vi "Get_ADAM_averages_client.vi"(6 "No of averages":i32=1, 7 "All Active Channels":bool, 9 "End time":dbl, 10 "Start time":dbl, 11 "ADAM Ch Names":string[](array[string])) -> (1 "Values":string[][](array[string]), 2 "Comments":string[](array[string]), 3 "Titles":string[](array[string]), 4 "Messages":string, 5 "DBL values":dbl[][](array[numeric]) format="%.2f")   [LabVIEW 2017]
doc: "This is an example of using features of the VI Server as a client. It shows how you might browse from one or more applications that may be exporting data from one or more data stations. \n\nThe example shows how to query a server for its list of exported VIs, how to get references to the VIs, and how call them with the Call By Reference function."
uses:
  Anemometry/Anemometry Sub Vis/Controls/Global_mode.ctl
  Sub VIs/ADAM Controls/Channel_names.ctl
  Anemometry/Anemometry Sub Vis/Globals/Preference_global.vi
panel:
  in  "vi type":refnum<vi>
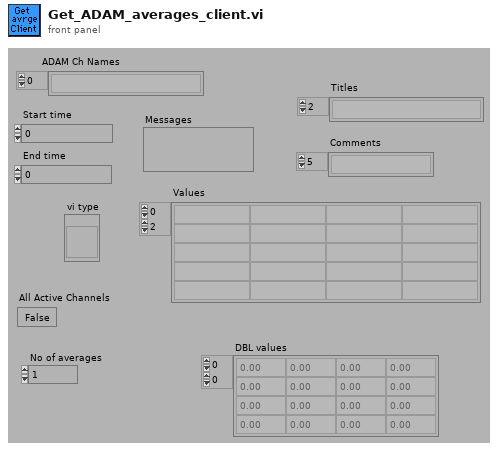
[diagram p1: front panel]
types:
  T1 = typedef "Global_mode.ctl" = enum16{"Read Global", "Load Global From File", "Write Global to File"}
  T2 = typedef "Channel_names.ctl" = enum16{"Active Only", "Active + Off", "All Channels"}
  T3 = typedef "Server_Comms.ctl" = enum16{"Server Link Healthy", "Do Not Link To Server"}
  T4 = typedef "Update_scan_value.ctl" = cluster{"Channel Name":string, "New Value":dbl}
  T5 = typedef "Ch_description_ADAM.ctl" = cluster{"Ch Name":string, "Type":T6, "Function":T7, "Ch State":T8, "Calibration type":T9, "A":dbl, "B":dbl, "C":dbl, "D":dbl, "Comments":string, "Address":T10, "String":string, "Duty":u16}
  T6 = typedef "Module_type_ADAM.ctl" = string
  T7 = typedef "Function_ADAM.ctl" = enum16{"Analogue Input", "Digital Input", "Event counter", "Event rate", "Analogue Output", "Digital Output", "Relay Output"}
  T8 = typedef "Channel_State.ctl" = enum16{"On", "Off", "Always On", "Always Off"}
  T9 = typedef "Calib_type_ADAM.ctl" = string
  T10 = typedef "Address.ctl" = cluster{"Main":i32, "Ch.":i32, "Sub":i32, "Port Name":string}
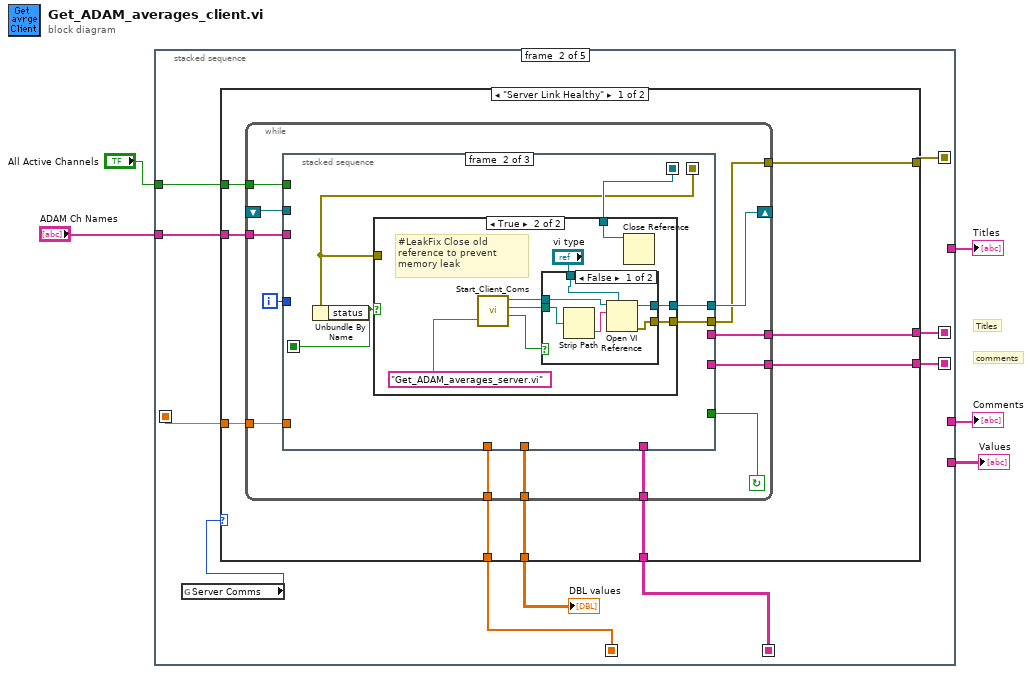
[diagram p0: block diagram]
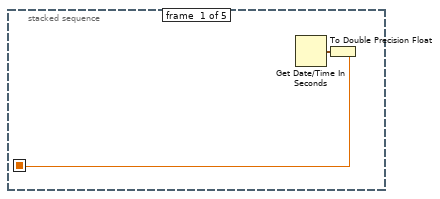
[diagram p2: hidden frame]
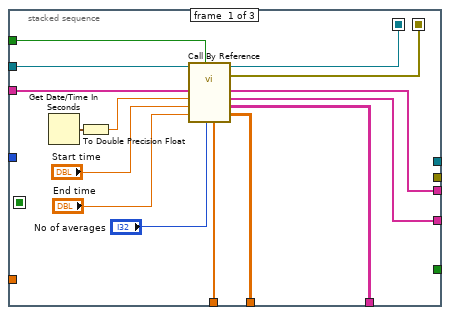
[diagram p3: hidden frame]
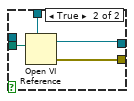
[diagram p5: hidden frame]
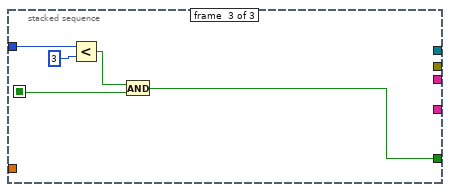
[diagram p6: hidden frame]
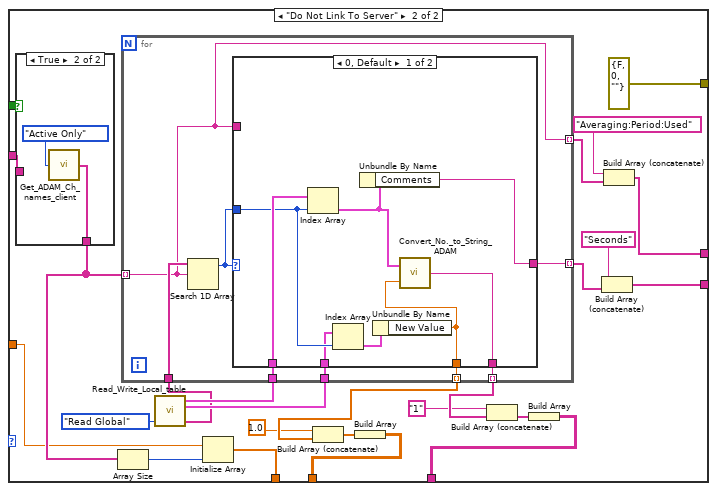
[diagram p7: hidden frame]
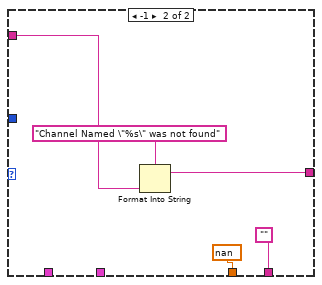
[diagram p9: hidden frame]
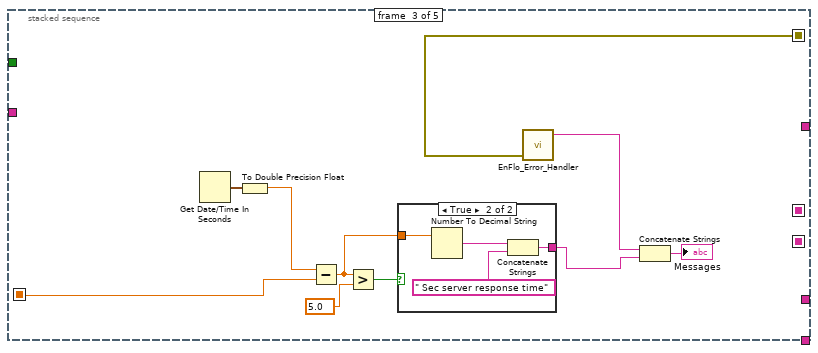
[diagram p10: hidden frame]
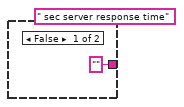
[diagram p11: hidden frame]
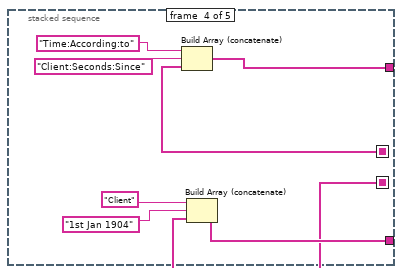
[diagram p12: hidden frame]
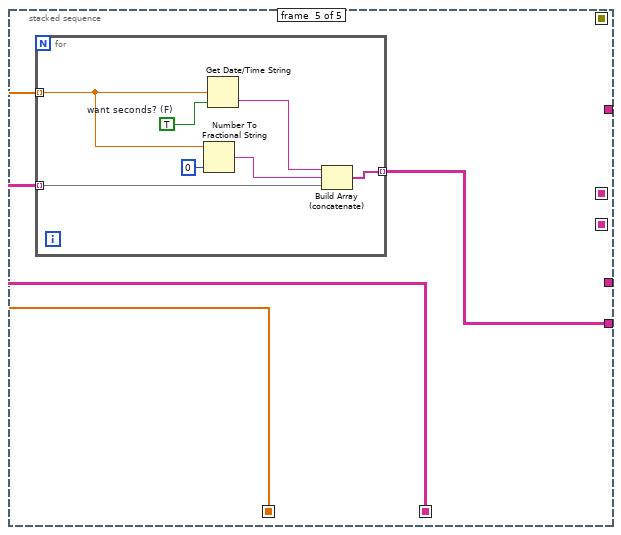
[diagram p13: hidden frame]
diagram:
  # "comments"
  # "Titles"
  n1 = stacked-sequence {
    seq-local: [_ w17 _ _ _] -> [_ _ _ w156 _]
    seq-local: [_ w8 _ _ _] -> [_ _ _ w149 _]
    seq-local: [_ w16 _ _ _] -> [_ _ _ _ w158]
    seq-local: [w7 _ _ _ _] -> [_ w15 w141 _ _]
    seq-local: [_ w14 _ _ _] -> [_ _ _ _ w159]
    seq-local: [_ w13 _ _ _] -> [_ _ w136 _ _]
    tunnel: [_ _ _ w154 _] -> w5
    tunnel: [_ _ _ w155 _] -> w4
    tunnel: [_ _ _ _ w157] -> w3
    tunnel: "ADAM Ch Names" -> [_ w10 _ _ _]
    tunnel: "All Active Channels" -> [_ w9 _ _ _]
    frame #0 {
      n2 = Get Date/Time In Seconds() -> (seconds since 1Jan1904=w6:timestamp)
      n3 = To Double Precision Float(number=w6) -> (double precision float=w7:dbl)
    }
    frame #1 {
      n4 = global read "Preference_global.vi" "Server Comms"() -> (w12:T3)
      n5 = case shown="\"Server Link Healthy\"" w12 {
        tunnel: [w26 w91] -> w17
        tunnel: [w25 w99] -> w16
        tunnel: w15 -> [w24 w89]
        tunnel: [w23 w105] -> w14
        tunnel: [w22 errorcluster {"status"=FALSE, "code"=0, "source"=""}] -> w13
        tunnel: [w21 w85] -> w11
        tunnel: w10 -> [w20 w100]
        tunnel: w9 -> [w19 w103]
        tunnel: [w18 w90] -> w8
        frame "Server Link Healthy" {
          n6 = while {
            tunnel: [w30] -> w22
            shift-left: _ -> [w34]
            shift-right: [w33] -> _
            tunnel: [w35] -> w23
            tunnel: w24 -> [w36]
            tunnel: [w37] -> w25
            tunnel: [w38] -> w18
            tunnel: [w39] -> w26
            tunnel: [w29] -> w21
            tunnel: w20 -> [w28]
            tunnel: w19 -> [w27]
            i -> [w32]
            stop <- w31 continue-if-true
            n7 = stacked-sequence {
              seq-local: [w44 _ _] -> [_ w58 _]
              seq-local: [w45 _ _] -> [_ w55 _]
              seq-local: [_ w57 _] -> [_ _ w81]
              tunnel: [w47 _ _] -> w39
              tunnel: [w52 _ _] -> w38
              tunnel: [w51 _ _] -> w37
              tunnel: w36 -> [_ _ _]
              tunnel: [w49 _ _] -> w35
              tunnel: w34 -> [w46 _ _]
              tunnel: [_ w59 _] -> w33
              tunnel: w32 -> [_ _ w82]
              tunnel: [_ _ w80] -> w31
              tunnel: [_ w56 _] -> w30
              tunnel: [w42 _ _] -> w29
              tunnel: w28 -> [w41 _ _]
              tunnel: w27 -> [w40 _ _]
              frame #0 {
                n8 = Get Date/Time In Seconds() -> (seconds since 1Jan1904=w43:timestamp)
                n9 = To Double Precision Float(number=w43) -> (double precision float=w53:dbl)
                n10 = call-by-ref "?"(reference=w46, "No of averages"="No of averages", "All Active Channels"=w40, "End time"="End time", "Start time"="Start time", "Clients time"=w53, "ADAM Ch Names"=w41) -> (reference out=w44:refnum<vi>, error out=w45:errorcluster, "DBL values"=w42:dbl[][], "Values"=w51:string[][], "Comments"=w52:string[], "Titles"=w47:string[], "Times"=w49:dbl[])  [unwired: 1 in]
              }
              frame #1 {
                n11 = Unbundle By Name(w55) -> ("status"=w57:bool)
                n12 = case shown="True" w57 {
                  tunnel: [w61 w65] -> w59
                  tunnel: w58 -> [w61 w62]
                  tunnel: [w60 w63] -> w56
                  tunnel: w55 -> [w60 _]
                  frame False {
                  }
                  frame True {
                    # "#LeakFix Close old reference to prevent memory leak"
                    n13 = call "Start_Client_Coms.vi"("VI name to run on server"="Get_ADAM_averages_server.vi") -> ("LabVIEW application reference"=w67:refnum<vi>, "Checked VI name"=w68:path, "Local Call"=w66:bool)  [unwired: 1 in, 1 out]
                    n14 = case shown="False" w66 {
                      tunnel: [w73 w79] -> w65
                      tunnel: "vi type" -> [w72 w78]
                      tunnel: w68 -> [w71 w77]
                      tunnel: w67 -> [w70 _]
                      tunnel: [w74 w76] -> w63
                      frame False {
                        n15 = Strip Path(path=w71) -> (name=w75:string)  [unwired: 1 out]
                        n16 = Open VI Reference(type specifier VI Refnum (for type only)=w72, application reference (local)=w70, vi path=w75) -> (vi reference=w73:refnum<vi>, error out=w74:errorcluster)  [unwired: 1 in, 2 out]
                      }
                      frame True {
                        n17 = Open VI Reference(type specifier VI Refnum (for type only)=w78, vi path=w77) -> (vi reference=w79:refnum<vi>, error out=w76:errorcluster)  [unwired: 1 in, 3 out]
                      }
                    }
                    n18 = Close Reference(reference=w62) -> ()  [unwired: 1 in, 1 out]
                  }
                }
              }
              frame #2 {
                n19 = Less?(x=w82, y=3) -> (x < y?=w83:bool)
                n20 = And(x=w83, y=w81) -> (x .and. y?=w80:bool)
              }
            }
          }
        }
        frame "Do Not Link To Server" {
          n21 = case shown="True" w103 {
            tunnel: [w110 w111] -> w102
            tunnel: w100 -> [w110 _]
            frame False {
            }
            frame True {
              n22 = call "Get_ADAM_Ch_names_client.vi"("Channel names set"=Channel_names."Active Only") -> ("Ch names"=w111:string[])
            }
          }
          n23 = Array Size(array=w102) -> (size(s)=w106:i32)
          n24 = call "Read_Write_Local_table.vi"("Mode"=Global_mode."Read Global") -> ("Ch Names"=w101:string[], "Ch Values Out"=w107:T4[], "Channels Descriptions Out"=w108:T5[])  [unwired: 2 in]
          n25 = for {
            tunnel: w101 -> [w117]
            tunnel: w102 -> [w116] mode=indexing
            tunnel: w108 -> [w119]
            tunnel: w107 -> [w118]
            tunnel: [w116] -> w92 mode=indexing
            tunnel: [w115] -> w96 mode=indexing
            tunnel: [w114] -> w98 mode=indexing
            tunnel: [w113] -> w88 mode=indexing
            n26 = Search 1D Array(1D array=w117, element=w116) -> (index of element=w120:i32)  [unwired: 1 out]
            n27 = case shown="0, Default" w120 {
              tunnel: w120 -> [w127 _]
              tunnel: w119 -> [w128 _]
              tunnel: w118 -> [w126 _]
              tunnel: w116 -> [_ w133]
              tunnel: [w123 w131] -> w115
              tunnel: [w122 ""] -> w114
              tunnel: [w121 nan ("New Value")] -> w113
              frame 0, Default {
                n28 = Index Array(array=w128, index=w127) -> (element=w124:T5)
                n29 = Index Array(array=w126, index=w127) -> (element=w125:T4)
                n30 = Unbundle By Name(w124) -> ("Comments"=w123:string)
                n31 = Unbundle By Name(w125) -> ("New Value"=w121:dbl)
                n32 = call "Convert_No._to_String_ADAM.vi"("Input number"=w121, "Ch Description"=w124) -> ("Output sting"=w122:string)
              }
              frame -1 {
                n33 = Format Into String(format string="Channel Named \"%s\" was not found" ("Format String"), w133) -> (resulting string=w131:string)  [unwired: 2 in, 1 out]
              }
            }
          }
          n34 = Initialize Array(w89, w106) -> (w105:dbl[])
          n35 = Build Array (concatenate)(1.0, w88) -> (w86:dbl[])
          n36 = Build Array(w86) -> (w85:dbl[][])
          n37 = Build Array (concatenate)("1", w98) -> (w97:string[])
          n38 = Build Array(w97) -> (w99:string[][])
          n39 = Build Array (concatenate)("Seconds", w96) -> (w90:string[])
          n40 = Build Array (concatenate)("Averaging:Period:Used", w92) -> (w91:string[])
        }
      }
      "DBL values" <- w11
    }
    frame #2 {
      n41 = Get Date/Time In Seconds() -> (seconds since 1Jan1904=w134:timestamp)
      n42 = To Double Precision Float(number=w134) -> (double precision float=w142:dbl)
      n43 = Subtract(x=w142, y=w141) -> (x-y=w138:dbl)
      n44 = Greater?(x=w138, y=5.0) -> (0:w139:bool)
      n45 = case shown="True" w139 {
        tunnel: w138 -> [_ w148]
        tunnel: ["" w145] -> w137
        frame False {
          (unwired) " sec server response time"
        }
        frame True {
          n46 = Number To Decimal String(number=w148) -> (decimal integer string=w146:string)  [unwired: 1 out]
          n47 = Concatenate Strings(w146, " Sec server response time") -> (w145:string)
        }
      }
      n48 = call "EnFlo_Error_Handler.vi"("error in (no error)"=w136) -> ("Email Message"=w135:string)  [unwired: 2 in, 2 out]
      n49 = Concatenate Strings(w135, w137) -> (→"Messages":string)
    }
    frame #3 {
      n50 = Build Array (concatenate)("Time:According:to", "Client:Seconds:Since", w156) -> (w154:string[])
      n51 = Build Array (concatenate)("Client" ("Comments"), "1st Jan 1904" ("Comments"), w149) -> (w155:string[])
    }
    frame #4 {
      n52 = for {
        tunnel: w159 -> [w161] mode=indexing
        tunnel: [w166] -> w157 mode=indexing
        tunnel: w158 -> [w165] mode=indexing
        w164 = TRUE  # want seconds? (F)
        n53 = Number To Fractional String(number=w161, precision (6)=i16 0) -> (F-format string=w160:string)  [unwired: 2 out]
        n54 = Get Date/Time String(seconds (now)=w161, want seconds? (F)=w164) -> (time string=w163:string)  [unwired: 2 out]
        n55 = Build Array (concatenate)(w163, w160, w165) -> (w166:string[])
      }
    }
  }
  "Titles" <- w5
  "Comments" <- w4
  "Values" <- w3
